vi "Test Customer with Phone Finishing Call Broadcasts Status.vi"(8 "error in (no error)":errorcluster, 11 "Customer With Phone Test In":refnum<class "Customer With Phone Test.lvclass">=refnum) -> (0 "error out":errorcluster, 3 "Customer With Phone Test Out":refnum<class "Customer With Phone Test.lvclass">)   [LabVIEW 2020, in "Customer With Phone Test.lvclass"]
uses:
  Customer With Phone Test.lvclass
  <vilib>/Astemes/Triarc Framework/Process/Process.lvclass
  Processes/People/Customers/Customer With Phone/Customer With Phone.lvclass
  C:/git/astemes-triarc-examples/source/Coffee Shop/Processes/People/Customers/Customer/Customer.lvclass
  C:/git/astemes-triarc-examples/source/Coffee Shop/Processes/People/Person/Person.lvclass
  C:/Program Files (x86)/National Instruments/LabVIEW 2020/vi.lib/Astemes/Triarc Framework/View/View.lvclass
  C:/Program Files (x86)/National Instruments/LabVIEW 2020/vi.lib/Astemes/Triarc Framework/Process/Process.lvclass
  C:/Program Files (x86)/National Instruments/LabVIEW 2020/vi.lib/Astemes/Triarc Framework/Base/Base.lvclass
  C:/Program Files (x86)/National Instruments/LabVIEW 2020/vi.lib/Astemes/Triarc Framework/Error Handler Interface/Error Handler Interface.lvclass
  C:/Program Files (x86)/National Instruments/LabVIEW 2020/vi.lib/Astemes/Triarc Framework/Logging/Logging.lvclass
  C:/git/astemes-triarc-examples/source/Coffee Shop/Processes/People/Process Job/Job Handler.lvclass
  C:/Program Files (x86)/National Instruments/LabVIEW 2020/vi.lib/Astemes/Triarc Framework/Async Handler/Async Handler.lvclass
  C:/git/astemes-triarc-examples/source/Coffee Shop/Processes/People/Customers/Customer With Phone/Customer With Phone.lvclass
  C:/Program Files (x86)/National Instruments/LabVIEW 2020/vi.lib/Astemes/Triarc Framework/Helper Loop/Helper Loop.lvclass
  0caa4622-e4aa-417c-bd7b-42e2749d9657.vi
  <vilib>/Astemes/Triarc Framework/Support/Broadcast Event Dequeuers.lvlib
  <vilib>/Astemes/LUnit/Test Case.lvclass
  C:/Program Files (x86)/National Instruments/LabVIEW 2020/vi.lib/Astemes/LUnit/Test Case.lvclass
  C:/Program Files (x86)/National Instruments/LabVIEW 2020/vi.lib/Astemes/LUnit/LUnit Runnable.lvclass
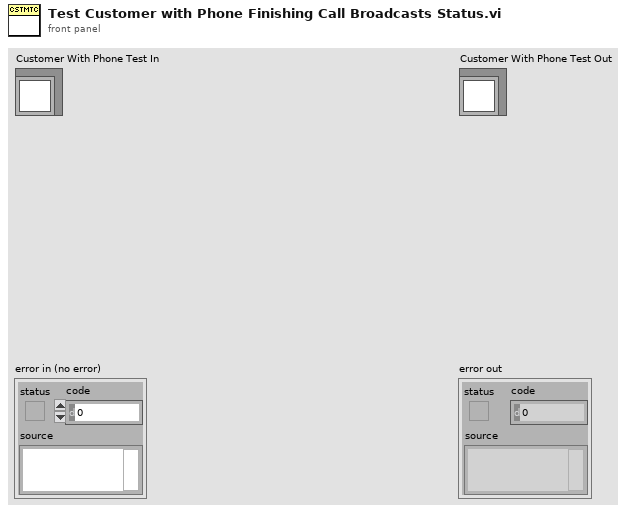
[diagram p1: front panel]
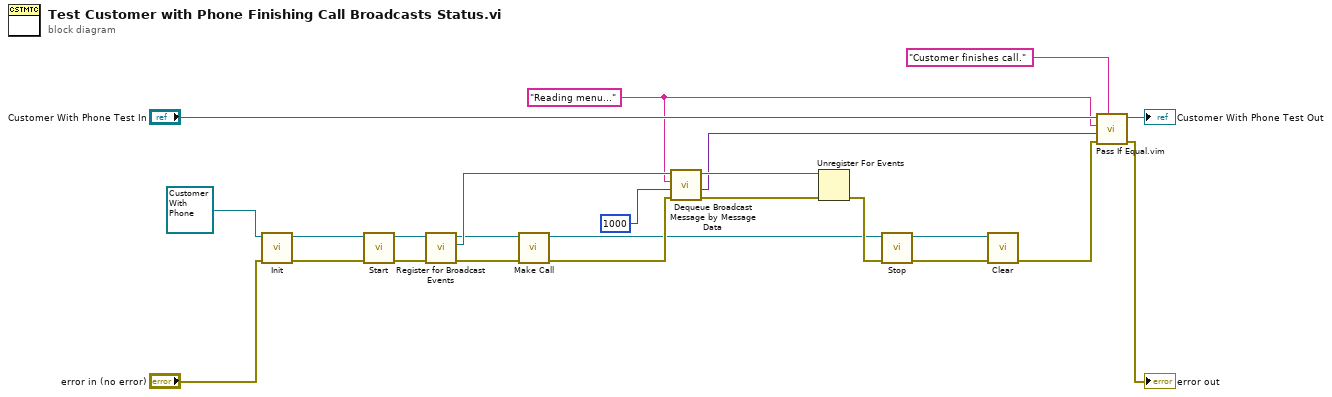
[diagram p0: block diagram]
diagram:
  w1 = "Reading menu..."
  n1 = call-dynamic "Init.vi"("error in (no error)"="error in (no error)", "View In"=refnum<class "Customer With Phone.lvclass"> refnum ("Customer With Phone.lvclass")) -> ("error out"=w24:errorcluster, "View Out"=w13:refnum<class "Customer With Phone.lvclass">)  [unwired: 8 in]
  n2 = call <vilib>:"Start.vi"("error in (no error)"=w24, "Process In"=w13) -> ("error out"=w16:errorcluster, "Process Out"=w18:refnum<class "Customer With Phone.lvclass">)  [unwired: 7 in, 1 out]
  n3 = call <vilib>:"Register for Broadcast Events.vi"("error in (no error)"=w16, "Process In"=w18) -> ("error out"=w17:errorcluster, "Event Registration Refnum Out"=w22:refnum<event-registration>, "Process Out"=w19:refnum<class "Customer With Phone.lvclass">)  [unwired: 7 in]
  n4 = call "Make Call.vi"("error in (no error)"=w17, "Customer With Phone In"=w19) -> ("error out"=w21:errorcluster, "Customer With Phone Out"=w20:refnum<class "Customer With Phone.lvclass">)  [unwired: 8 in]
  n5 = call <vilib>:"Dequeue Broadcast Message by Message Data.vi"("error in (no error)"=w21, "Timeout (-1)"=1000, "Message Data"=w1, "Event Registration Refnum"=w22) -> ("error out"=w4:errorcluster, "Message Data"=w2:variant, "Event Registration Refnum Out"=w5:refnum<event-registration>)  [unwired: 3 in, 2 out]
  n6 = Unregister For Events(event registration refnum=w5, error in=w4) -> (error out=w23:errorcluster)
  n7 = call <vilib>:"Stop.vi"("error in (no error)"=w23, "Process In"=w20) -> ("error out"=w15:errorcluster, "Process Out"=w14:refnum<class "Customer With Phone.lvclass">)  [unwired: 7 in, 1 out]
  n8 = call-dynamic "Clear.vi"("error in (no error)"=w15, "View In"=w14) -> ("error out"=w7:errorcluster)  [unwired: 9 in]
  n9 = call "Pass If Equal.vim"("Description"="Customer finishes call.", "error in (no error)"=w7, "Actual"=w2, "Expected"=w1, "LUnit Test Case In"="Customer With Phone Test In") -> ("error out"=→"error out":errorcluster, "LUnit Test Case Out"=→"Customer With Phone Test Out":refnum<class "Test Case.lvclass">)  [unwired: 5 in]
